vi "LOC subGetFileExtension.vi"(1 "FileName":string) -> (0 "FileExtension (no dot)":string)   [LabVIEW 2020, in "Localization_Tools.lvlib"]
uses:
  Localization_Tools.lvlib
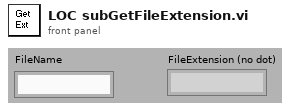
[diagram p1: front panel]
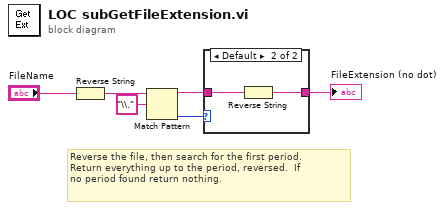
[diagram p0: block diagram]
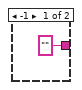
[diagram p2: hidden frame]
diagram:
  # "Reverse the file, then search for the first period.\nReturn everything up to the period, reversed.  If\nno period found return nothing."
  n1 = Reverse String(1:"FileName") -> (0:w5:string)
  n2 = Match Pattern(string=w5, regular expression="\\.") -> (before substring=w3:string, offset past match=w1:i32)  [unwired: 1 in, 2 out]
  n3 = case shown="Default" w1 {
    tunnel: w3 -> [_ w9]
    tunnel: ["" w8] -> w2
    frame -1 {
    }
    frame Default {
      n4 = Reverse String(1:w9) -> (0:w8:string)
    }
  }
  "FileExtension (no dot)" <- w2
